vi "SMAC.vi"() -> ()   [LabVIEW 2019, in "Class 2.lvclass"]
uses:
  Class 2.lvclass
panel:
  out "POS INI":i32=895
  out "SM READ":string="TP\r\n895\r\n>" caption="LECTURA DEL SMAC"
  in  "stop":bool
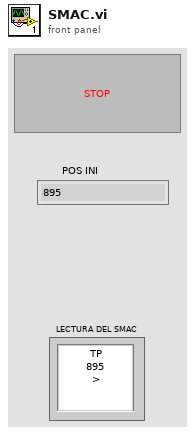
[diagram p1: front panel]
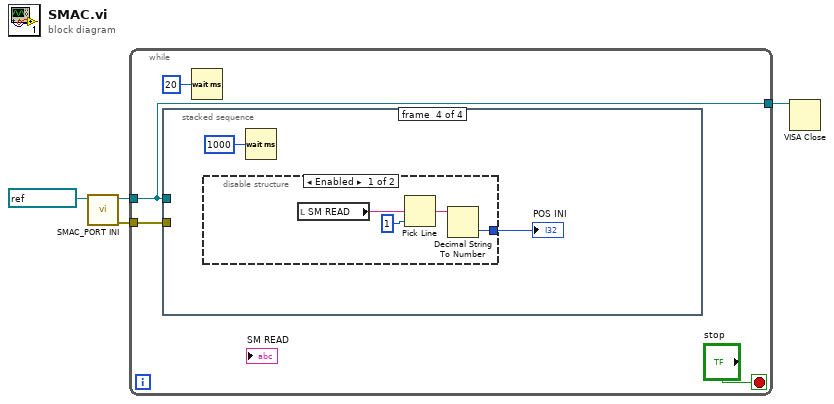
[diagram p0: block diagram]
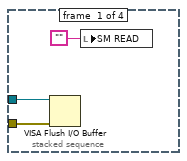
[diagram p2: hidden frame]
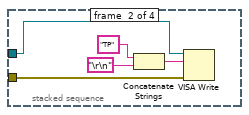
[diagram p3: hidden frame]
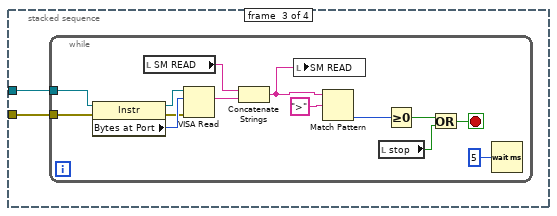
[diagram p4: hidden frame]
diagram:
  n1 = call "SMAC_PORT INI.vi"("VISA Refnum in"=refnum<visa-resource-name> "COM19" ("VISA resource name")) -> ("error out"=w2:errorcluster, "VISA resource name out"=w3:refnum<visa-resource-name>)  [unwired: 9 in]
  n2 = while {
    tunnel: w3 -> [w5]
    tunnel: w2 -> [w6]
    tunnel: [w5] -> w1
    stop <- "stop" stop-if-true
    n3 = stacked-sequence {
      tunnel: w5 -> [w9 w13 w18 _]
      tunnel: w6 -> [w10 w12 w17 _]
      frame #0 {
        n4 = VISA Flush I/O Buffer(VISA resource name=w9, error in (no error)=w10) -> ()  [unwired: 1 in, 2 out]
        n5 = local write "SM READ"("") -> ()
      }
      frame #1 {
        n6 = Concatenate Strings("TP" ("write buffer"), "\r\n") -> (w14:string)
        n7 = VISA Write(VISA resource name=w13, write buffer=w14, error in (no error)=w12) -> ()  [unwired: 3 out]
      }
      frame #2 {
        n8 = while {
          tunnel: w18 -> [w28]
          tunnel: w17 -> [w27]
          stop <- w21 stop-if-true
          n9 = property class="Instr"(reference=w28, error in=w27) -> (reference out=w30:refnum<visa-resource-name>, error out=w31:errorcluster, "Bytes at Port"=w32:u32)
          n10 = local read "SM READ"() -> (w26:string)
          n11 = VISA Read(VISA resource name=w30, byte count=w32, error in (no error)=w31) -> (read buffer=w29:string)  [unwired: 3 out]
          n12 = Concatenate Strings(w26, w29) -> (w23:string)
          n13 = local write "SM READ"(w23) -> ()
          n14 = Match Pattern(string=w23, regular expression=">") -> (offset past match=w25:i32)  [unwired: 1 in, 3 out]
          n15 = local read "stop"() -> (w20:bool)
          n16 = Greater Or Equal To 0?(x=w25) -> (x >= 0?=w22:bool)
          n17 = Or(x=w22, y=w20) -> (x .or. y?=w21:bool)
          n18 = Wait (ms)(milliseconds to wait=u32 5) -> ()  [unwired: 1 out]
        }
      }
      frame #3 {
        n19 = disable-structure shown="Enabled" {
          disable-tunnel: [w35 _] -> w34
          frame Enabled {
            n20 = local read "SM READ"() -> (w36:string)
            n21 = Pick Line(multi-line string=w36, line index=1) -> (output string=w37:string)  [unwired: 1 in]
            n22 = Decimal String To Number(string=w37) -> (number=w35:i32)  [unwired: 2 in, 1 out]
          }
          frame Disabled {
          }
        }
        "POS INI" <- w34
        n23 = Wait (ms)(milliseconds to wait=u32 1000) -> ()  [unwired: 1 out]
      }
    }
    n24 = Wait (ms)(milliseconds to wait=u32 20) -> ()  [unwired: 1 out]
  }
  n25 = VISA Close(VISA resource name=w1) -> ()  [unwired: 1 in, 1 out]
